vi "create completed tour report.vi"(1 "report format":T1, 2 "tour number":u64, 3 "completed_tour":T2) -> (0 "completed tour (log paragraph)":string)   [LabVIEW 2020, in "main.lvlib"]
doc: "Converts the knight tour to a paragraph of text to be logged to file."
uses:
  main.lvlib
  core/core_data/completed_tour.ctl
  core/core_data/chessboard_index.ctl
  core/core_data/tour type (enum).ctl
  report format.ctl
  <vilib>/Utility/error.llb/Clear Errors.vi
  convert--tour to string (minimal format).vi
  PTRL/string/Number (U64) to comma delimited string.vi
  convert--tour to string (chessboard format).vi
  PTRL/string/Number (DBL) to comma delimited string.vi
  core/core_data/core_data.lvlib
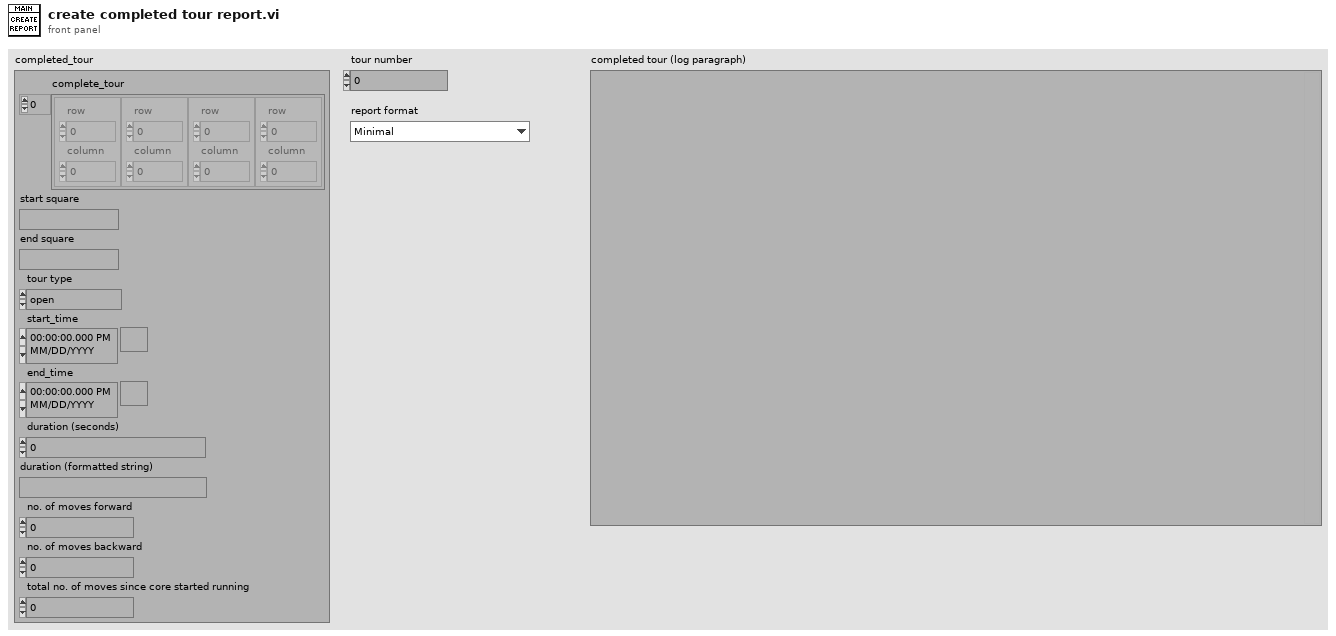
[diagram p1: front panel]
types:
  T1 = typedef "main.lvlib/report format.ctl" = enum16{"Minimal", "Detailed"}
  T2 = typedef "core.lvlib/core_data.lvlib/completed_tour.ctl" = cluster{"complete_tour":T3[], "start square":string, "end square":string, "tour type":T4, "start_time":timestamp, "end_time":timestamp, "duration (seconds)":dbl, "duration (formatted string)":string, "no. of moves forward":u64, "no. of moves backward":u64, "total no. of moves since core started running":u64}
  T3 = typedef "core.lvlib/core_data.lvlib/chessboard_index.ctl" = cluster{"row":u8, "column":u8}
  T4 = typedef "core.lvlib/core_data.lvlib/tour type (enum).ctl" = enum16{"open", "closed"}
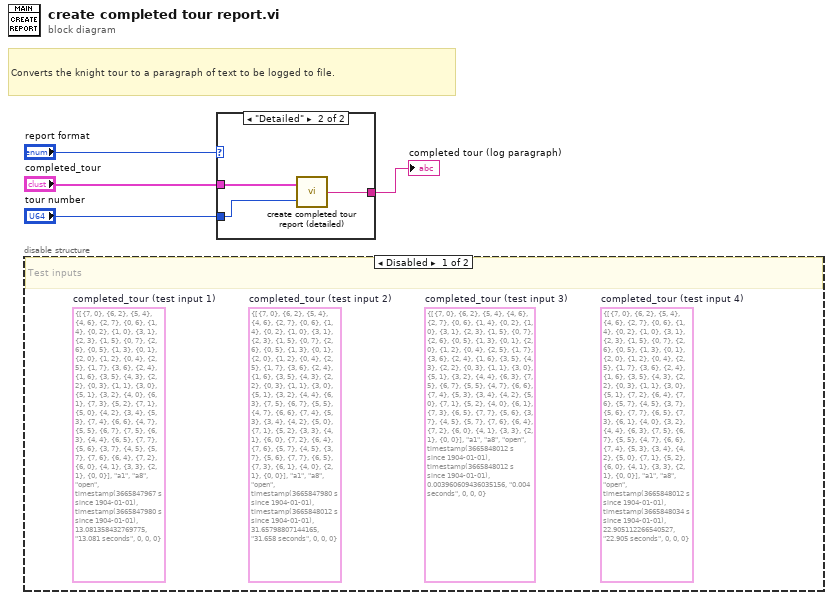
[diagram p0: block diagram]
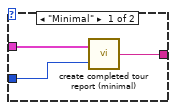
[diagram p2: hidden frame]
diagram:
  # "Converts the knight tour to a paragraph of text to be logged to file."
  n1 = disable-structure shown="Disabled" {
    frame Disabled {
      (unwired) T2 {"complete_tour"=[{"row"=7, "column"=0}, {"row"=6, "column"=2}, {"row"=5, "column"=4}, {"row"=4, "column"=6}, {"row"=2, "column"=7}, {"row"=0, "column"=6}, {"row"=1, "column"=4}, {"row"=0, "column"=2}, {"row"=1, "column"=0}, {"row"=3, "column"=1}, {"row"=2, "column"=3}, {"row"=1, "column"=5}, {"row"=0, "column"=7}, {"row"=2, "column"=6}, {"row"=0, "column"=5}, {"row"=1, "column"=3}, {"row"=0, "column"=1}, {"row"=2, "column"=0}, {"row"=1, "column"=2}, {"row"=0, "column"=4}, {"row"=2, "column"=5}, {"row"=1, "column"=7}, {"row"=3, "column"=6}, {"row"=2, "column"=4}, {"row"=1, "column"=6}, {"row"=3, "column"=5}, {"row"=4, "column"=3}, {"row"=2, "column"=2}, {"row"=0, "column"=3}, {"row"=1, "column"=1}, {"row"=3, "column"=0}, {"row"=5, "column"=1}, {"row"=7, "column"=2}, {"row"=6, "column"=4}, {"row"=7, "column"=6}, {"row"=5, "column"=7}, {"row"=4, "column"=5}, {"row"=3, "column"=7}, {"row"=5, "column"=6}, {"row"=7, "column"=7}, {"row"=6, "column"=5}, {"row"=7, "column"=3}, {"row"=6, "column"=1}, {"row"=4, "column"=0}, {"row"=3, "column"=2}, {"row"=4, "column"=4}, {"row"=6, "column"=3}, {"row"=7, "column"=5}, {"row"=6, "column"=7}, {"row"=5, "column"=5}, {"row"=4, "column"=7}, {"row"=6, "column"=6}, {"row"=7, "column"=4}, {"row"=5, "column"=3}, {"row"=3, "column"=4}, {"row"=4, "column"=2}, {"row"=5, "column"=0}, {"row"=7, "column"=1}, {"row"=5, "column"=2}, {"row"=6, "column"=0}, {"row"=4, "column"=1}, {"row"=3, "column"=3}, {"row"=2, "column"=1}, {"row"=0, "column"=0}], "start square"="a1", "end square"="a8", "tour type"=enum."open", "start_time"=timestamp(3665848012.019379 s since 1904-01-01), "end_time"=timestamp(3665848034.9244914 s since 1904-01-01), "duration (seconds)"=22.905112266540527, "duration (formatted string)"="22.905 seconds", "no. of moves forward"=0, "no. of moves backward"=0, "total no. of moves since core started running"=0}  # completed_tour (test input 4)
      (unwired) T2 {"complete_tour"=[{"row"=7, "column"=0}, {"row"=6, "column"=2}, {"row"=5, "column"=4}, {"row"=4, "column"=6}, {"row"=2, "column"=7}, {"row"=0, "column"=6}, {"row"=1, "column"=4}, {"row"=0, "column"=2}, {"row"=1, "column"=0}, {"row"=3, "column"=1}, {"row"=2, "column"=3}, {"row"=1, "column"=5}, {"row"=0, "column"=7}, {"row"=2, "column"=6}, {"row"=0, "column"=5}, {"row"=1, "column"=3}, {"row"=0, "column"=1}, {"row"=2, "column"=0}, {"row"=1, "column"=2}, {"row"=0, "column"=4}, {"row"=2, "column"=5}, {"row"=1, "column"=7}, {"row"=3, "column"=6}, {"row"=2, "column"=4}, {"row"=1, "column"=6}, {"row"=3, "column"=5}, {"row"=4, "column"=3}, {"row"=2, "column"=2}, {"row"=0, "column"=3}, {"row"=1, "column"=1}, {"row"=3, "column"=0}, {"row"=5, "column"=1}, {"row"=3, "column"=2}, {"row"=4, "column"=4}, {"row"=6, "column"=3}, {"row"=7, "column"=5}, {"row"=6, "column"=7}, {"row"=5, "column"=5}, {"row"=4, "column"=7}, {"row"=6, "column"=6}, {"row"=7, "column"=4}, {"row"=5, "column"=3}, {"row"=3, "column"=4}, {"row"=4, "column"=2}, {"row"=5, "column"=0}, {"row"=7, "column"=1}, {"row"=5, "column"=2}, {"row"=4, "column"=0}, {"row"=6, "column"=1}, {"row"=7, "column"=3}, {"row"=6, "column"=5}, {"row"=7, "column"=7}, {"row"=5, "column"=6}, {"row"=3, "column"=7}, {"row"=4, "column"=5}, {"row"=5, "column"=7}, {"row"=7, "column"=6}, {"row"=6, "column"=4}, {"row"=7, "column"=2}, {"row"=6, "column"=0}, {"row"=4, "column"=1}, {"row"=3, "column"=3}, {"row"=2, "column"=1}, {"row"=0, "column"=0}], "start square"="a1", "end square"="a8", "tour type"=enum."open", "start_time"=timestamp(3665848012.0154185 s since 1904-01-01), "end_time"=timestamp(3665848012.019379 s since 1904-01-01), "duration (seconds)"=0.003960609436035156, "duration (formatted string)"="0.004 seconds", "no. of moves forward"=0, "no. of moves backward"=0, "total no. of moves since core started running"=0}  # completed_tour (test input 3)
      (unwired) T2 {"complete_tour"=[{"row"=7, "column"=0}, {"row"=6, "column"=2}, {"row"=5, "column"=4}, {"row"=4, "column"=6}, {"row"=2, "column"=7}, {"row"=0, "column"=6}, {"row"=1, "column"=4}, {"row"=0, "column"=2}, {"row"=1, "column"=0}, {"row"=3, "column"=1}, {"row"=2, "column"=3}, {"row"=1, "column"=5}, {"row"=0, "column"=7}, {"row"=2, "column"=6}, {"row"=0, "column"=5}, {"row"=1, "column"=3}, {"row"=0, "column"=1}, {"row"=2, "column"=0}, {"row"=1, "column"=2}, {"row"=0, "column"=4}, {"row"=2, "column"=5}, {"row"=1, "column"=7}, {"row"=3, "column"=6}, {"row"=2, "column"=4}, {"row"=1, "column"=6}, {"row"=3, "column"=5}, {"row"=4, "column"=3}, {"row"=2, "column"=2}, {"row"=0, "column"=3}, {"row"=1, "column"=1}, {"row"=3, "column"=0}, {"row"=5, "column"=1}, {"row"=3, "column"=2}, {"row"=4, "column"=4}, {"row"=6, "column"=3}, {"row"=7, "column"=5}, {"row"=6, "column"=7}, {"row"=5, "column"=5}, {"row"=4, "column"=7}, {"row"=6, "column"=6}, {"row"=7, "column"=4}, {"row"=5, "column"=3}, {"row"=3, "column"=4}, {"row"=4, "column"=2}, {"row"=5, "column"=0}, {"row"=7, "column"=1}, {"row"=5, "column"=2}, {"row"=3, "column"=3}, {"row"=4, "column"=1}, {"row"=6, "column"=0}, {"row"=7, "column"=2}, {"row"=6, "column"=4}, {"row"=7, "column"=6}, {"row"=5, "column"=7}, {"row"=4, "column"=5}, {"row"=3, "column"=7}, {"row"=5, "column"=6}, {"row"=7, "column"=7}, {"row"=6, "column"=5}, {"row"=7, "column"=3}, {"row"=6, "column"=1}, {"row"=4, "column"=0}, {"row"=2, "column"=1}, {"row"=0, "column"=0}], "start square"="a1", "end square"="a8", "tour type"=enum."open", "start_time"=timestamp(3665847980.3574305 s since 1904-01-01), "end_time"=timestamp(3665848012.0154185 s since 1904-01-01), "duration (seconds)"=31.65798807144165, "duration (formatted string)"="31.658 seconds", "no. of moves forward"=0, "no. of moves backward"=0, "total no. of moves since core started running"=0}  # completed_tour (test input 2)
      (unwired) T2 {"complete_tour"=[{"row"=7, "column"=0}, {"row"=6, "column"=2}, {"row"=5, "column"=4}, {"row"=4, "column"=6}, {"row"=2, "column"=7}, {"row"=0, "column"=6}, {"row"=1, "column"=4}, {"row"=0, "column"=2}, {"row"=1, "column"=0}, {"row"=3, "column"=1}, {"row"=2, "column"=3}, {"row"=1, "column"=5}, {"row"=0, "column"=7}, {"row"=2, "column"=6}, {"row"=0, "column"=5}, {"row"=1, "column"=3}, {"row"=0, "column"=1}, {"row"=2, "column"=0}, {"row"=1, "column"=2}, {"row"=0, "column"=4}, {"row"=2, "column"=5}, {"row"=1, "column"=7}, {"row"=3, "column"=6}, {"row"=2, "column"=4}, {"row"=1, "column"=6}, {"row"=3, "column"=5}, {"row"=4, "column"=3}, {"row"=2, "column"=2}, {"row"=0, "column"=3}, {"row"=1, "column"=1}, {"row"=3, "column"=0}, {"row"=5, "column"=1}, {"row"=3, "column"=2}, {"row"=4, "column"=0}, {"row"=6, "column"=1}, {"row"=7, "column"=3}, {"row"=5, "column"=2}, {"row"=7, "column"=1}, {"row"=5, "column"=0}, {"row"=4, "column"=2}, {"row"=3, "column"=4}, {"row"=5, "column"=3}, {"row"=7, "column"=4}, {"row"=6, "column"=6}, {"row"=4, "column"=7}, {"row"=5, "column"=5}, {"row"=6, "column"=7}, {"row"=7, "column"=5}, {"row"=6, "column"=3}, {"row"=4, "column"=4}, {"row"=6, "column"=5}, {"row"=7, "column"=7}, {"row"=5, "column"=6}, {"row"=3, "column"=7}, {"row"=4, "column"=5}, {"row"=5, "column"=7}, {"row"=7, "column"=6}, {"row"=6, "column"=4}, {"row"=7, "column"=2}, {"row"=6, "column"=0}, {"row"=4, "column"=1}, {"row"=3, "column"=3}, {"row"=2, "column"=1}, {"row"=0, "column"=0}], "start square"="a1", "end square"="a8", "tour type"=enum."open", "start_time"=timestamp(3665847967.276072 s since 1904-01-01), "end_time"=timestamp(3665847980.3574305 s since 1904-01-01), "duration (seconds)"=13.081358432769775, "duration (formatted string)"="13.081 seconds", "no. of moves forward"=0, "no. of moves backward"=0, "total no. of moves since core started running"=0}  # completed_tour (test input 1)
      # "Test inputs"
    }
    frame Enabled {
    }
  }
  n2 = case shown="\"Detailed\"" "report format" {
    tunnel: "completed_tour" -> [w7 w10]
    tunnel: "tour number" -> [w6 w9]
    tunnel: [w5 w8] -> w1
    frame "Minimal" {
      n3 = call "create completed tour report (minimal).vi"("tour number"=w6, "completed_tour"=w7) -> ("completed tour (log paragraph)"=w5:string)
    }
    frame "Detailed" {
      n4 = call "create completed tour report (detailed).vi"("tour number"=w9, "completed_tour"=w10) -> ("completed tour (log paragraph)"=w8:string)
    }
  }
  "completed tour (log paragraph)" <- w1
